vi "Cell V Set All.vi"(7 "Box ID":u8, 8 "error in (no error)":errorcluster, 10 "Voltage":dbl, 11 "ENET in":refnum<class "ENET_BS120x.lvclass">) -> (0 "error out":errorcluster, 3 "ENET out":refnum<class "ENET_BS120x.lvclass">)   [LabVIEW 2021, in "BS120x Driver.lvlib" / "ENET_BS120x.lvclass"]
uses:
  ENET_BS120x.lvclass
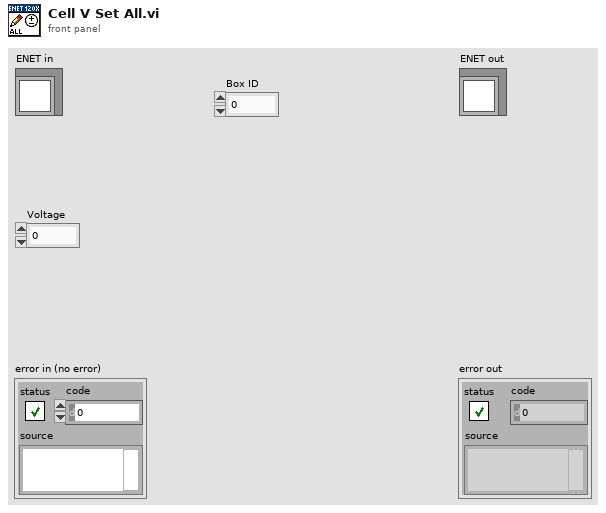
[diagram p1: front panel]
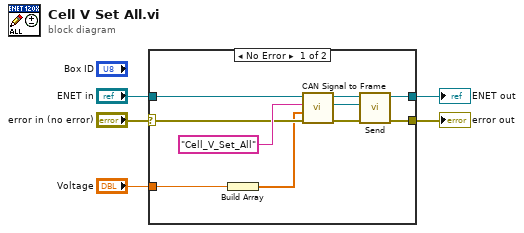
[diagram p0: block diagram]
diagram:
  n1 = case shown="No Error" "error in (no error)" {
    selector: "error in (no error)" -> [w10 w16]
    tunnel: [w11 w16] -> w5
    tunnel: "Voltage" -> [w9 _]
    tunnel: "ENET in" -> [w7 w17]
    tunnel: [w6 w17] -> w1
    frame No Error {
      n2 = Build Array(w9) -> (w8:dbl[])
      n3 = call "CAN Signal to Frame.vi"("error in (no error)"=w10, "Data Array"=w8, "Frame"="Cell_V_Set_All", "ENET in"=w7) -> ("error out"=w12:errorcluster, "Data"=w13:refnum<class "Data.lvclass">, "ENET out"=w14:refnum<class "ENET_BS120x.lvclass">)  [unwired: 5 in]
      n4 = call "Send.vi"("error in (no error)"=w12, "Data"=w13, "ENET in"=w14) -> ("error out"=w11:errorcluster, "ENET out"=w6:refnum<class "ENET_BS120x.lvclass">)  [unwired: 7 in]
    }
    frame Error {
    }
  }
  "error out" <- w5
  "ENET out" <- w1
